vi "Scope Measurement.vi"(0 "Scope Reference":refnum<k15>, 5 "Scope Channels":string, 11 "error in (no error)":errorcluster, 13 "Scope Timeout (s)":dbl) -> (4 "Measured Output Voltage":cluster{dbl[], dbl[]}, 6 "Measured Load Current":cluster{dbl[], dbl[]}, 15 "error out":errorcluster)   [LabVIEW 2020, in "LDO Load Transient.lvlib"]
uses:
  LDO Load Transient.lvlib
  <instrlib>/niScope/Acquire/Fetch/niScope Multi Fetch Cluster.vi
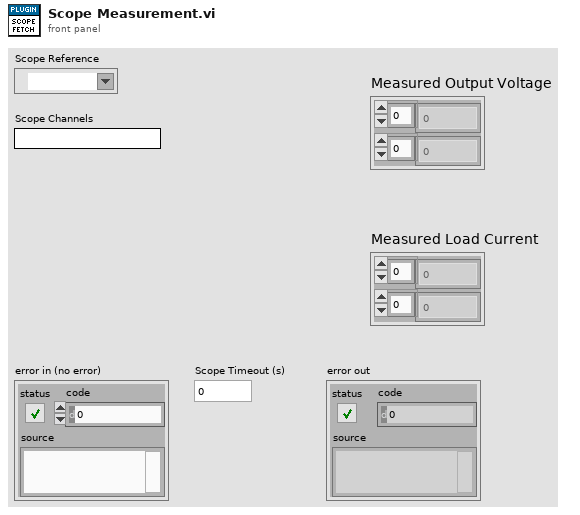
[diagram p1: front panel]
types:
  T1 = cluster{"relativeInitialX":dbl, "xIncrement":dbl, "wfm":dbl[]}[]
  T2 = cluster{"relativeInitialX":dbl, "xIncrement":dbl, "wfm":dbl[]}
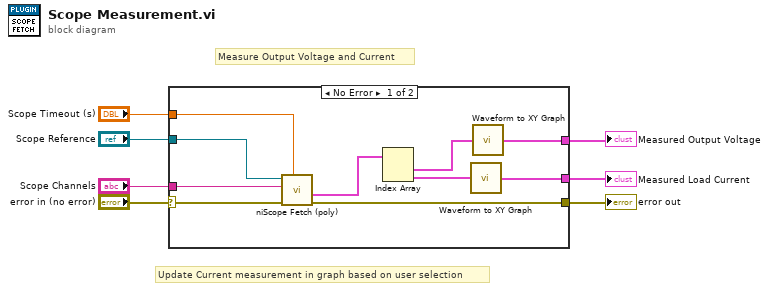
[diagram p0: block diagram]
diagram:
  # "Update Current measurement in graph based on user selection"
  # "Measure Output Voltage and Current"
  n1 = case shown="No Error" "error in (no error)" {
    selector: "error in (no error)" -> [w13 w18]
    tunnel: "Scope Reference" -> [w17 _]
    tunnel: "Scope Timeout (s)" -> [w15 _]
    tunnel: [w14 w18] -> w5
    tunnel: "Scope Channels" -> [w12 _]
    tunnel: [w10 _] -> w2
    tunnel: [w9 _] -> w1
    frame No Error {
      n2 = call-poly <instrlib>:"niScope Fetch (poly).vi"("timeout"=w15, "error in"=w13, "channels"=w12, "instrument handle"=w17) -> ("error out"=w14:errorcluster, "waveform"=w16:T1)  [unwired: 4 in, 2 out]
      n3 = Index Array(array=w16) -> (element #1=w8:T2, element #2=w11:T2)  [unwired: 2 in]
      n4 = call "Waveform to XY Graph.vi"("Measure Load Current"=w11) -> ("Scope Waveform"=w10:cluster{dbl[], dbl[]})  [unwired: 14 in]
      n5 = call "Waveform to XY Graph.vi"("Measure Load Current"=w8) -> ("Scope Waveform"=w9:cluster{dbl[], dbl[]})  [unwired: 14 in]
    }
    frame Error {
    }
  }
  "error out" <- w5
  "Measured Load Current" <- w2
  "Measured Output Voltage" <- w1
